vi "sine.vi"() -> ()   [LabVIEW 2019]
panel:
  in  "stop":bool
  out "Waveform Graph":dynamicdata(graph)
  in  "frequency":dbl(knob) scale=0.0..50.0
  in  "Knob":dbl(knob) scale=0.0..10.0
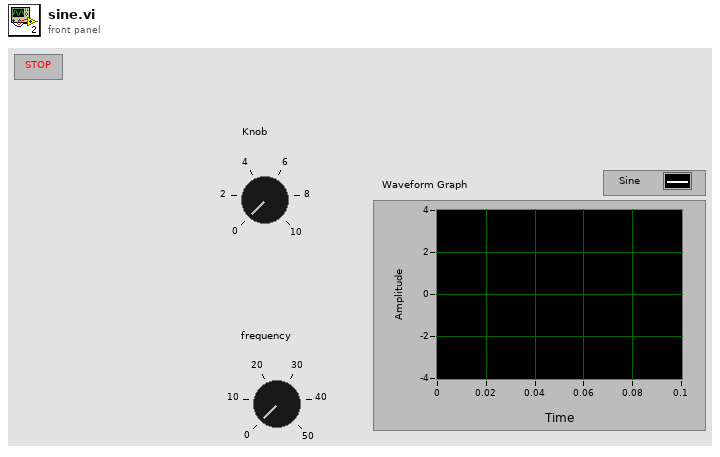
[diagram p1: front panel]
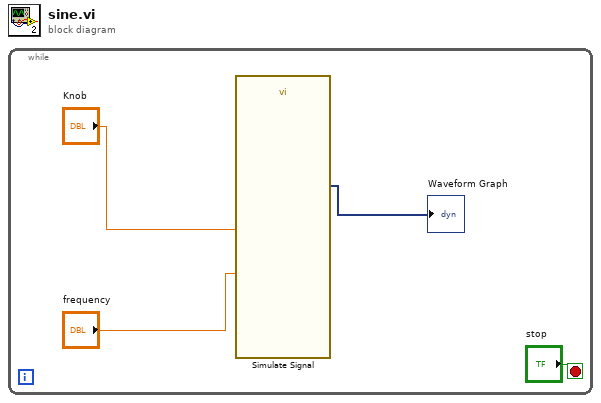
[diagram p0: block diagram]
diagram:
  n1 = while {
    stop <- "stop" stop-if-true
    n2 = call "Simulate Signal"("Frequency"="frequency", "Amplitude"="Knob") -> ("Sine"=→"Waveform Graph":dynamicdata)  [unwired: 12 in, 1 out]
  }
